vi "FP Demo.vi"() -> ()   [LabVIEW 2020]
panel:
  in  "Save Button 2":bool
  in  "Save Button":bool
  in  "Print Button":bool
  out "Waveform Chart":dbl(graph)
  out "String":string
  # "Title ...."
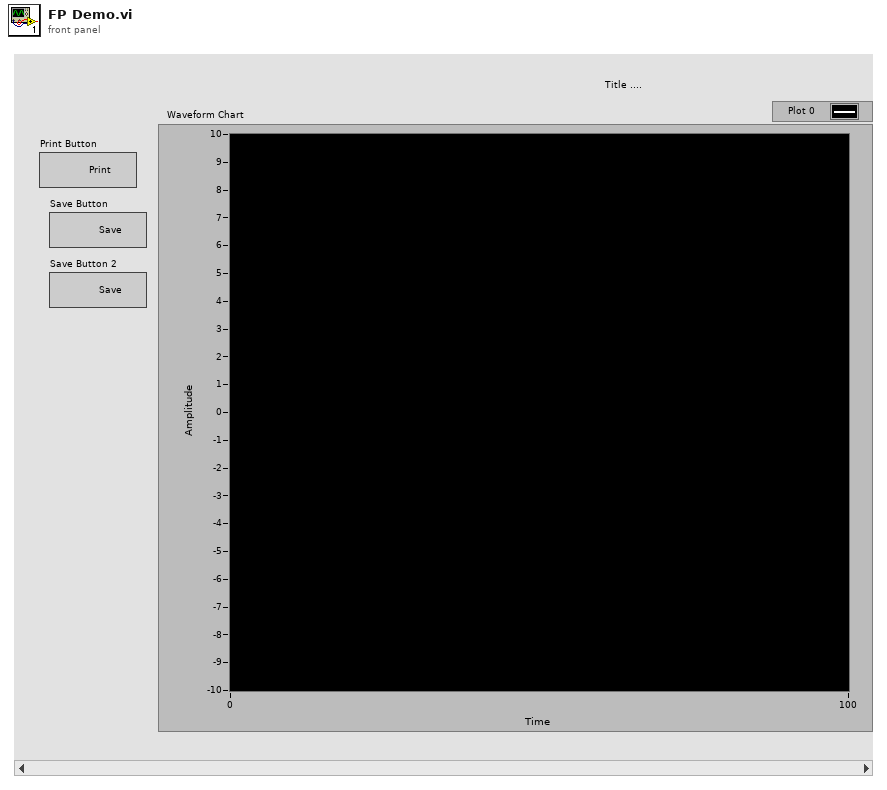
[diagram p1: front panel]
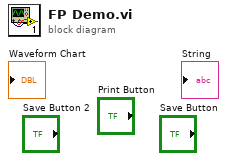
[diagram p0: block diagram]
diagram:
